vi "Scaled Quadrant Vector.vi"(9 "Y Positive":bool, 10 "X Positive":bool, 11 "Scale Mag":dbl) -> (1 "Combined":i32, 2 "Negated Y":i32, 3 "Scaled Sign Vector":cluster{"X":dbl, "Y":dbl})   [LabVIEW 2020]
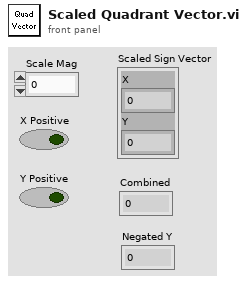
[diagram p1: front panel]
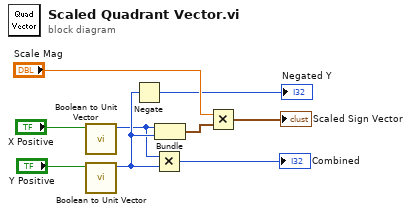
[diagram p0: block diagram]
diagram:
  n1 = call "Boolean to Unit Vector.vi"("Y Positive"="X Positive") -> ("Numeric"=w4:i32)  [unwired: 10 in]
  n2 = call "Boolean to Unit Vector.vi"("Y Positive"="Y Positive") -> ("Numeric"=w6:i32)  [unwired: 10 in]
  n3 = Negate(x=w6) -> (-x=→"Negated Y":i32)
  n4 = Multiply(x=w4, y=w6) -> (x*y=→"Combined":i32)
  n5 = Bundle("Numeric"=w4, "Numeric"=w6) -> (w1:cluster{"Numeric":i32, "Numeric":i32})  [unwired: 1 in]
  n6 = Multiply(x="Scale Mag", y=w1) -> (x*y=→"Scaled Sign Vector":cluster{"Numeric":dbl, "Numeric":dbl})
